vi "remove_negative_num.vi"(1 "Array in":dbl[][](array[numeric])) -> (0 "Array out":dbl[][](array[numeric]))   [LabVIEW 2019]
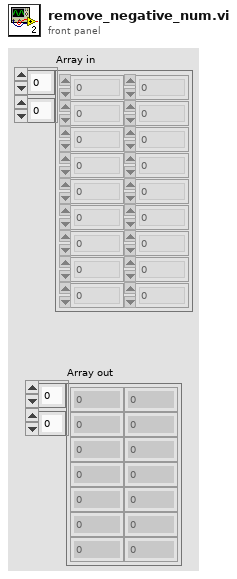
[diagram p1: front panel]
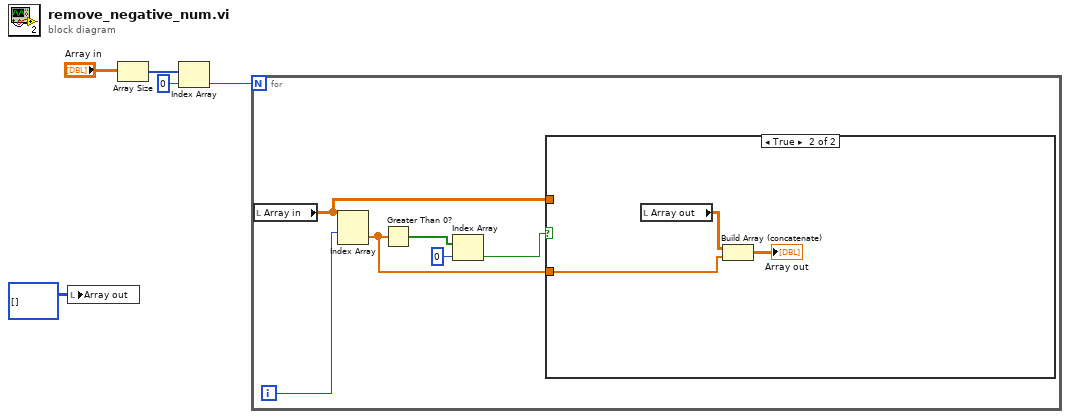
[diagram p0: block diagram]
diagram:
  n1 = local write "Array out"(i32[][] [] ("Array out")) -> ()
  n2 = Array Size(array="Array in") -> (size(s)=w4:i32[])
  n3 = Index Array(array=w4, index=0) -> (element=w2:i32)
  n4 = for {
    N: w2 -> [_]
    i -> [w11]
    n5 = local read "Array in"() -> (w10:dbl[][])
    n6 = Index Array(array=w10, index (row)=w11) -> (element=w6:dbl[])  [unwired: 1 in]
    n7 = Greater Than 0?(x=w6) -> (x > 0?=w9:bool[])
    n8 = Index Array(array=w9, index=0) -> (element=w8:bool)
    n9 = case shown="True" w8 {
      tunnel: w10 -> [_ _]
      tunnel: w6 -> [_ w12]
      frame False {
      }
      frame True {
        n10 = local read "Array out"() -> (w13:dbl[][])
        n11 = Build Array (concatenate)(w13, w12) -> (→"Array out":dbl[][])
      }
    }
  }
